vi "Do.vi"(8 "error in (no error)":errorcluster, 10 "Actor in":refnum<class "Actor.lvclass">, 11 "GetRecord Msg":refnum<class "GetRecord Msg.lvclass">) -> (0 "error out":errorcluster, 2 "Actor out":refnum<class "Actor.lvclass">)   [LabVIEW 2025, in "Task_Abstr.lvlib" / "GetRecord Msg.lvclass"]
doc: "This VI delivers the message to the actor by calling the appropriate method(s) on the actor."
uses:
  GetRecord Msg.lvclass
  GetRecord Msg.lvclass/GetRecord Msg.ctl
  9ef47adc-f318-494c-9b8b-6df3216d6863.vi
  Task_Abstr/Task_Abstr.lvclass
  <vilib>/ActorFramework/Actor/Actor.lvclass
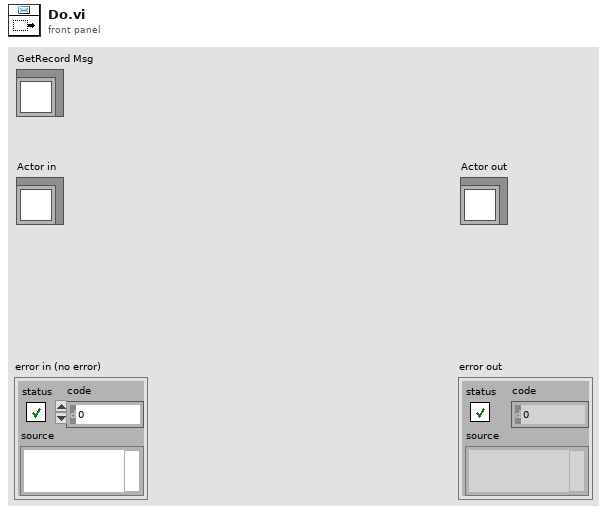
[diagram p1: front panel]
types:
  T1 = typedef "Task_Abstr.lvlib/Task_Abstr.lvclass/WaveformData.ctl" = cluster{"StartTime":timestamp, "StopTime":timestamp, "Waveform":waveform(dbl)[]}
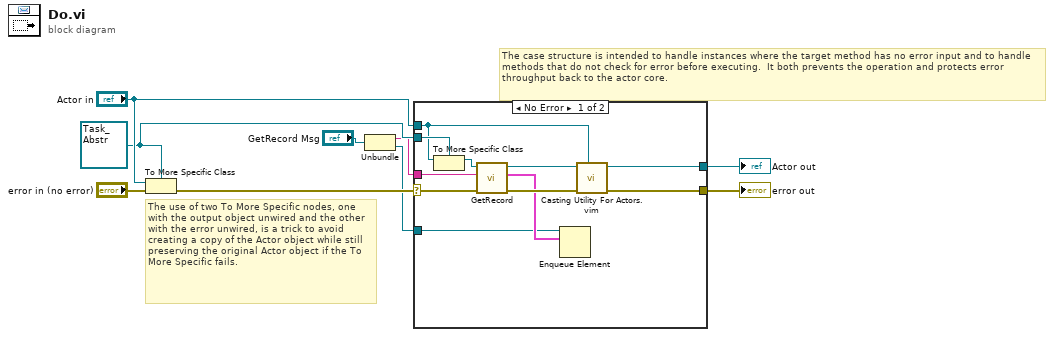
[diagram p0: block diagram]
diagram:
  w3 = refnum<class "Task_Abstr.lvclass"> refnum ("Actor in")
  # "The use of two To More Specific nodes, one with the output object unwired and the other with the error unwired, is a trick to avoid creating a copy of the Actor object while still preserving the original Actor object if the To More Specific fails."
  # "The case structure is intended to handle instances where the target method has no error input and to handle methods that do not check for error before executing.  It both prevents the operation and protects error throughput back to the actor core."
  n1 = To More Specific Class(target class=w3, reference="Actor in", error in="error in (no error)") -> (error out=w7:errorcluster)  [unwired: 1 out]
  n2 = Unbundle("GetRecord Msg") -> (w2:string, w1:refnum<queue>)
  n3 = case shown="No Error" w7 {
    selector: w7 -> [w20 w22]
    tunnel: [w14 w22] -> w6
    tunnel: [w15 w21] -> w5
    tunnel: "Actor in" -> [w17 w21]
    tunnel: w3 -> [w18 _]
    tunnel: w2 -> [w12 _]
    tunnel: w1 -> [w10 _]
    frame No Error {
      n4 = To More Specific Class(target class=w18, reference=w17) -> (specific class reference=w19:refnum<class "Task_Abstr.lvclass">)  [unwired: 1 in, 1 out]
      n5 = call-dynamic "GetRecord.vi"("error in (no error)"=w20, "Label"=w12, "Task_Abstr in"=w19) -> ("error out"=w13:errorcluster, "WaveformData"=w11:T1, "Task_Abstr out"=w16:refnum<class "Task_Abstr.lvclass">)  [unwired: 6 in]
      n6 = Enqueue Element(queue=w10, element=w11) -> ()  [unwired: 2 in, 3 out]
      n7 = call "Casting Utility For Actors.vim"("type"=w17, "error in (no error)"=w13, "Actor in"=w16) -> ("error out"=w14:errorcluster, "Actor out"=w15:refnum<class "Actor.lvclass">)  [unwired: 7 in]
    }
    frame Error {
      # "If type check fails, pass the original object out again."
    }
  }
  "error out" <- w6
  "Actor out" <- w5
